vi "Pump Close Selection.vi"(8 "error in (no error)":errorcluster, 11 "Pump Settings In":T1={"Output Device"=enum."Default", "Masterflex"={"VISA resource name"="", "Simulated?"=FALSE, "Pump Number"=0.0, "Reverse?"=FALSE}, "Ismatech"={"VISA resource name"="", "Simulated?"=FALSE, "Pump Number"=0.0, "Reverse?"=FALSE}, "Ismatech 3 Channel Settings"={"VISA resource name"="", "Pump Number"=1, "Channel Number"=0, "Simulated?"=TRUE, "Reverse?"=FALSE}, "VICI Settings"={"VISA resource name"="", "Pump ID"="", "Pump Head Vol"=0.0, "Reverse?"=FALSE, "Simulated?"=FALSE}, "Tacmina Settings"={"Analog DAQ Task"="", "Digital DAQ Task"=""}, "KNF SIMDOS Settings"={"VISA resource name"="", "Simulated?"=FALSE}, "ASIA Pump C"={"ASIA Pump #"=0, "channel"=0, "Simulated"=FALSE}, "FLOM Settings"={"VISA resource name"="", "Simulated?"=FALSE, "Pump Number"=0.0}, "SSI PR/LD Settings"={"VISA resource name"="", "Simulated?"=FALSE}, "SSI P40 Settings"={"VISA resource name"="", "Simulated?"=FALSE}, "Masterflex 75211 Settings"={"Analog DAQ Task"="", "Digital DAQ Task"=""}} {"Ismatech 3 Channel Settings"."Channel Number" min=0 max=3; "Ismatech 3 Channel Settings"."Pump Number" min=1; "Masterflex"."Pump Number" min=1.0 max=20.0 step=1.0; "Ismatech"."Pump Number" min=1.0 max=20.0 step=1.0; "ASIA Pump C"."channel" min=-1 max=1 step=1}) -> (0 "error out":errorcluster, 1 "Connection Error":bool, 3 "Pump Settings Out":T1={"Output Device"=enum."Default", "Masterflex"={"VISA resource name"="", "Simulated?"=FALSE, "Pump Number"=0.0, "Reverse?"=FALSE}, "Ismatech"={"VISA resource name"="", "Simulated?"=FALSE, "Pump Number"=0.0, "Reverse?"=FALSE}, "Ismatech 3 Channel Settings"={"VISA resource name"="", "Pump Number"=1, "Channel Number"=0, "Simulated?"=TRUE, "Reverse?"=FALSE}, "VICI Settings"={"VISA resource name"="", "Pump ID"="", "Pump Head Vol"=0.0, "Reverse?"=FALSE, "Simulated?"=FALSE}, "Tacmina Settings"={"Analog DAQ Task"="", "Digital DAQ Task"=""}, "KNF SIMDOS Settings"={"VISA resource name"="", "Simulated?"=FALSE}, "ASIA Pump C"={"ASIA Pump #"=0, "channel"=0, "Simulated"=FALSE}, "FLOM Settings"={"VISA resource name"="", "Simulated?"=FALSE, "Pump Number"=0.0}, "SSI PR/LD Settings"={"VISA resource name"="", "Simulated?"=FALSE}, "SSI P40 Settings"={"VISA resource name"="", "Simulated?"=FALSE}, "Masterflex 75211 Settings"={"Analog DAQ Task"="", "Digital DAQ Task"=""}} {"Ismatech 3 Channel Settings"."Channel Number" min=0 max=3; "Ismatech 3 Channel Settings"."Pump Number" min=1; "Masterflex"."Pump Number" min=1.0 max=20.0 step=1.0; "Ismatech"."Pump Number" min=1.0 max=20.0 step=1.0; "ASIA Pump C"."channel" min=-1 max=1 step=1})   [LabVIEW 2018, in "Pump Module.lvlib" / "Pump Module Engine.lvlib"]
uses:
  Measure Instrument/Pump Module Engine.lvlib
  Measure Instrument/Pump Settings Cluster.ctl
  Measure Instrument/PID 2 Output Enum.ctl
  Masterflex 7550-30/Controls/Settings Cluster.ctl
  Ismatec ISM 831C/Controls/Ismatech ISM831C Settings Cluster.ctl
  Ismatec 78001/Ismatec 4083.ctl
  VICI M50 Party Mode/Settings Cluster.ctl
  Tacmina QI/Tacmina QI DAQ Setting.ctl
  KNF Pump/Settings Cluster plus SIMDOS.ctl
  ASIA Pump/Pump Settings.ctl
  FLOM Pump/Settings Cluster.ctl
  SSI PR Class/SSI PR or LD Settings Cluster.ctl
  Masterflex 75211/Masterflex 75211 DAQ Setting.ctl
  Ismatec ISM 831C/Ismatec ISM 831C.lvlib
  Masterflex 7550-30/Masterflex 7550-30.lvlib
  VICI M50 Party Mode/VICI M6 M50 Party Mode.lvlib
  Tacmina QI/Tacmina QI.lvlib
  KNF Pump/KNF SIMDOS.lvlib
  ASIA Pump.lvlib
  FLOM Pump/FLOM Pump.lvlib
  SSI PR Class/SSI PR or LD Pump.lvlib
  Masterflex 75211/Masterflex 75211.lvlib
  SSI PR Class/SSI P40 Pump.lvlib
  Pump Module.lvlib
  Ismatec 78001/Ismatec 4308.lvlib
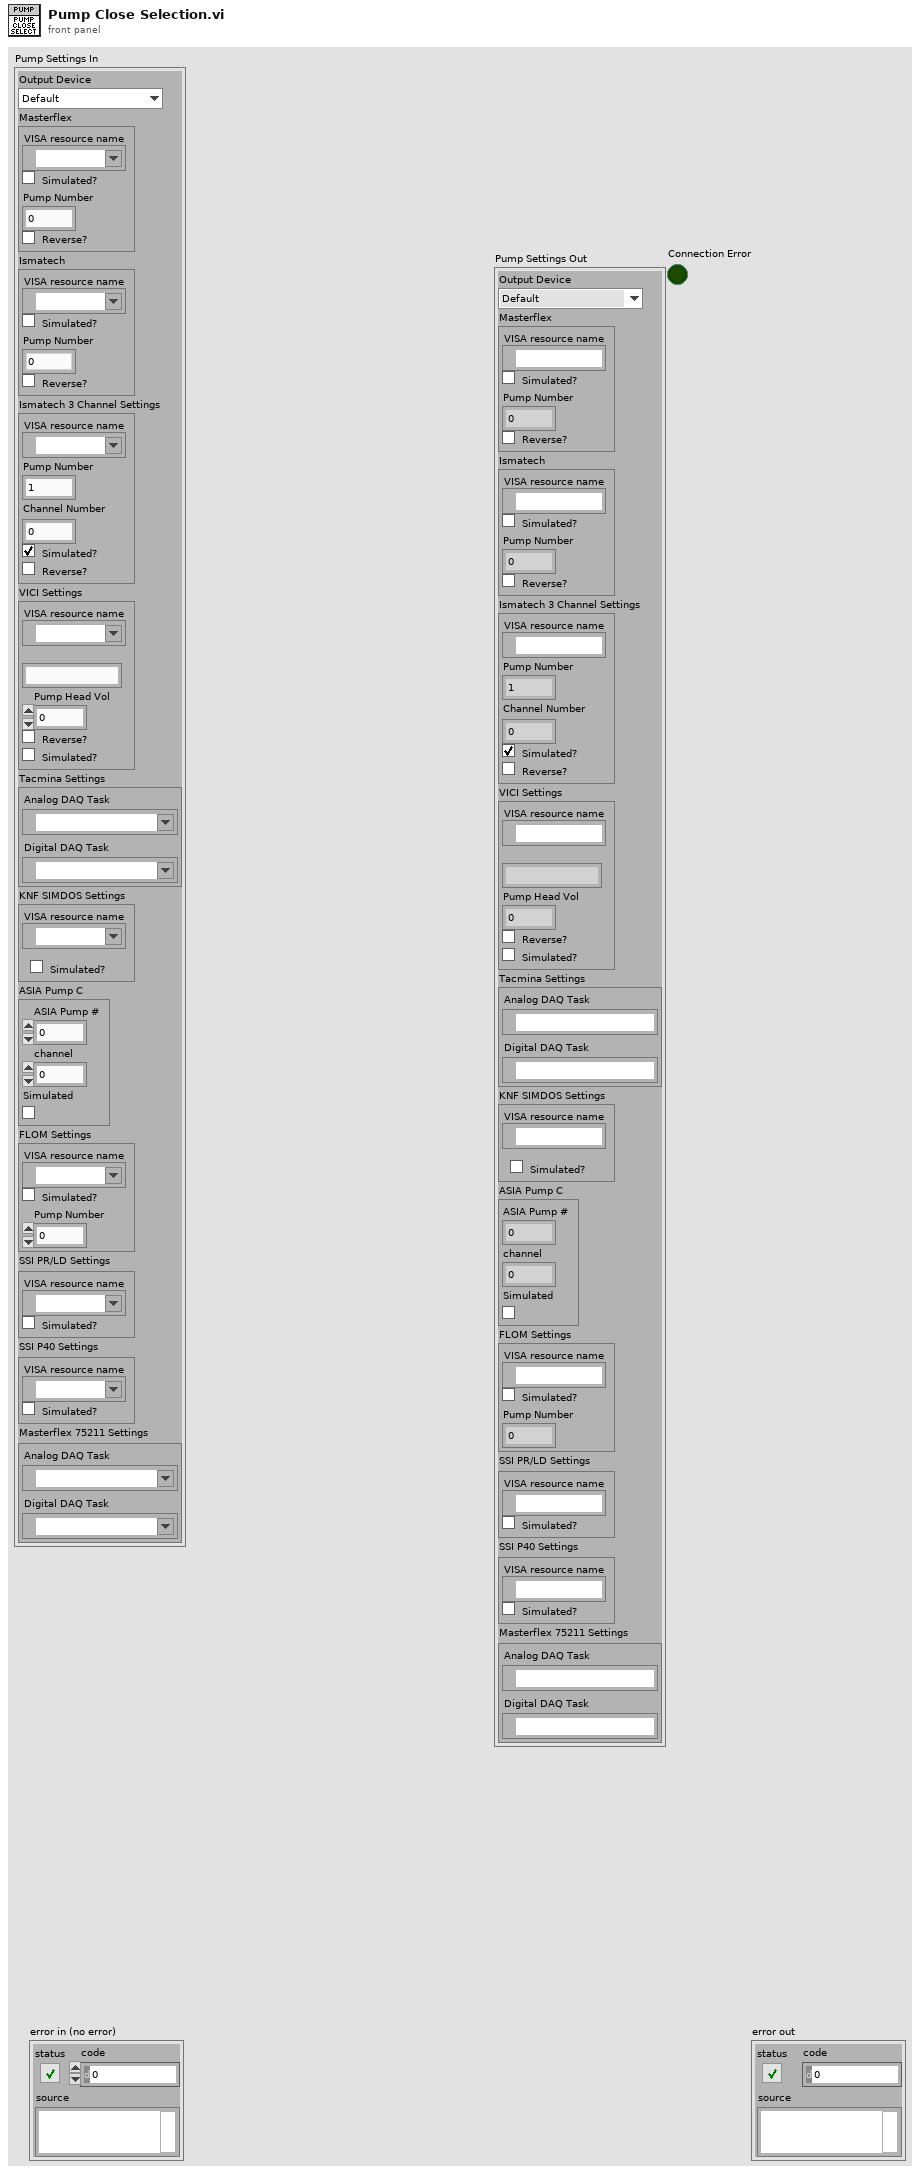
[diagram p1: front panel]
types:
  T1 = typedef "Pump Module.lvlib/Pump Settings Cluster.ctl" = cluster{"Output Device":T2, "Masterflex":T3, "Ismatech":T4, "Ismatech 3 Channel Settings":T5, "VICI Settings":T6, "Tacmina Settings":T7, "KNF SIMDOS Settings":T8, "ASIA Pump C":T9, "FLOM Settings":T10, "SSI PR/LD Settings":T11, "SSI P40 Settings":T11, "Masterflex 75211 Settings":T12}
  T2 = typedef "PID 2 Output Enum.ctl" = enum16{"Default", "Ismatec ISM 4308", "Ismatec ISM 831C", "Masterflex 7550-30", "VICI", "Tacmina QI", "KNF SIMDOS", "ASIA Type C", "FLOM UI-22-11", "SSI PR/LD", "SSI P40", "Masterflex 75211-70"}
  T3 = typedef "Masterflex 7550-30.lvlib/Settings Cluster.ctl" = cluster{"VISA resource name":refnum<visa-resource-name>, "Simulated?":bool, "Pump Number":dbl, "Reverse?":bool}
  T4 = typedef "Ismatec ISM 831C.lvlib/Ismatech ISM831C Settings Cluster.ctl" = cluster{"VISA resource name":refnum<visa-resource-name>, "Simulated?":bool, "Pump Number":dbl, "Reverse?":bool}
  T5 = typedef "Ismatec 4308.lvlib/Ismatec 4083.ctl" = cluster{"VISA resource name":refnum<visa-resource-name>, "Pump Number":i16, "Channel Number":i16, "Simulated?":bool, "Reverse?":bool}
  T6 = typedef "VICI M6 M50 Party Mode.lvlib/Settings Cluster.ctl" = cluster{"VISA resource name":refnum<visa-resource-name>, "Pump ID":string, "Pump Head Vol":dbl, "Reverse?":bool, "Simulated?":bool}
  T7 = typedef "Tacmina QI.lvlib/Tacmina QI DAQ Setting.ctl" = cluster{"Analog DAQ Task":refnum<k21>, "Digital DAQ Task":refnum<k21>}
  T8 = typedef "KNF SIMDOS.lvlib/Settings Cluster plus SIMDOS.ctl" = cluster{"VISA resource name":refnum<visa-resource-name>, "Simulated?":bool}
  T9 = typedef "ASIA Pump.lvlib/Pump Settings.ctl" = cluster{"ASIA Pump #":i32, "channel":i32, "Simulated":bool}
  T10 = typedef "FLOM Pump.lvlib/Settings Cluster.ctl" = cluster{"VISA resource name":refnum<visa-resource-name>, "Simulated?":bool, "Pump Number":dbl}
  T11 = typedef "SSI PR or LD Pump.lvlib/SSI PR or LD Settings Cluster.ctl" = cluster{"VISA resource name":refnum<visa-resource-name>, "Simulated?":bool}
  T12 = typedef "Masterflex 75211.lvlib/Masterflex 75211 DAQ Setting.ctl" = cluster{"Analog DAQ Task":refnum<k21>, "Digital DAQ Task":refnum<k21>}
  T13 = typedef "SSI P40 Pump.lvlib/SSI P40 Settings Cluster.ctl" = cluster{"VISA resource name":refnum<visa-resource-name>, "Simulated?":bool}
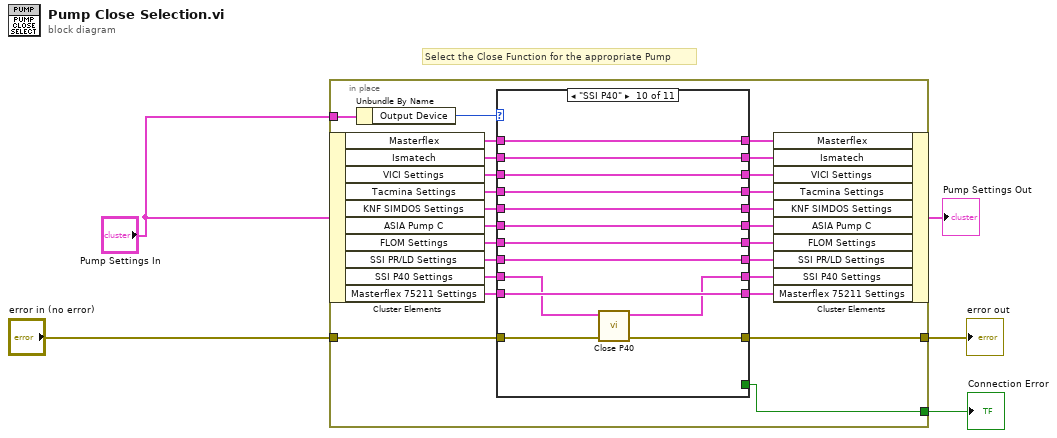
[diagram p0: block diagram]
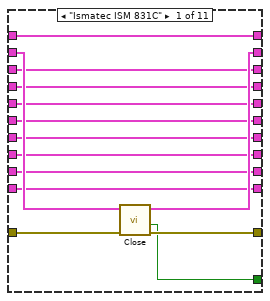
[diagram p2: hidden frame]
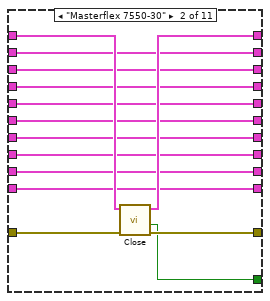
[diagram p3: hidden frame]
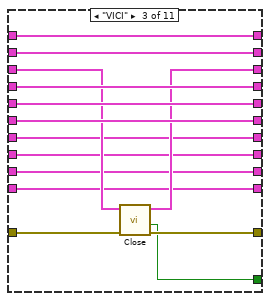
[diagram p4: hidden frame]
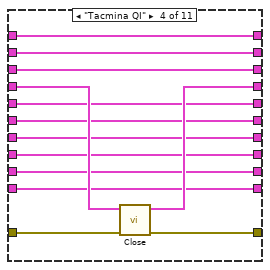
[diagram p5: hidden frame]
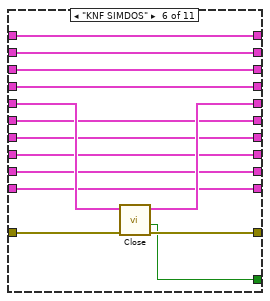
[diagram p7: hidden frame]
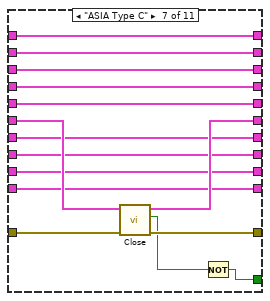
[diagram p8: hidden frame]
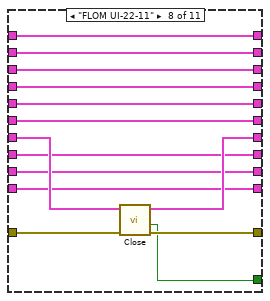
[diagram p9: hidden frame]
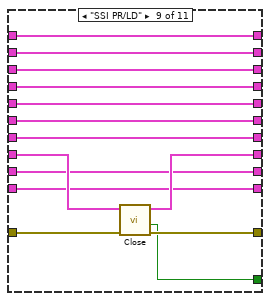
[diagram p10: hidden frame]
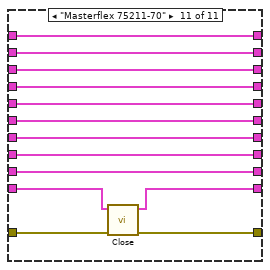
[diagram p11: hidden frame]
diagram:
  # "Select the Close Function for the appropriate Pump"
  n1 = in-place {
    in-place-border: "error in (no error)" -> [w29]
    in-place-border: [w28] -> w4
    in-place-border: "Pump Settings In" -> [w27]
    in-place-border: [w26] -> w3
    n2 = in-place-cluster #1("Pump Settings In") -> ("Masterflex"=w25:T3, "Ismatech"=w24:T4, "VICI Settings"=w23:T6, "Tacmina Settings"=w22:T7, "KNF SIMDOS Settings"=w21:T8, "ASIA Pump C"=w20:T9, "FLOM Settings"=w19:T10, "SSI PR/LD Settings"=w18:T11, "SSI P40 Settings"=w7:T11, "Masterflex 75211 Settings"=w9:T12)
    n3 = Unbundle By Name(w27) -> ("Output Device"=w30:T2)
    n4 = case shown="\"SSI P40\"" w30 {
      tunnel: w25 -> [w40 w58 w69 w82 w96 w110 w123 w139 w153 w165 w178]
      tunnel: [w40 w57 w69 w82 w96 w110 w123 w139 w153 w165 w178] -> w17
      tunnel: w24 -> [w42 w55 w70 w83 w95 w109 w122 w138 w152 w163 w177]
      tunnel: [w44 w56 w71 w84 w94 w106 w124 w132 w145 w164 w169] -> w28
      tunnel: w29 -> [w43 w54 w72 w85 w94 w107 w125 w133 w146 w164 w170]
      tunnel: [w41 w55 w70 w83 w95 w109 w122 w138 w152 w163 w177] -> w16
      tunnel: [w39 w53 w68 w81 w93 w108 w121 w136 w150 w162 w176] -> w14
      tunnel: w22 -> [w39 w53 w68 w80 w93 w108 w121 w136 w150 w162 w176]
      tunnel: [w38 w52 w67 w79 w92 w105 w120 w135 w149 w161 w175] -> w13
      tunnel: w21 -> [w38 w52 w67 w79 w92 w104 w120 w135 w149 w161 w175]
      tunnel: w20 -> [w37 w51 w66 w78 w91 w103 w119 w134 w148 w160 w174]
      tunnel: [w37 w51 w66 w78 w91 w103 w118 w134 w148 w160 w174] -> w12
      tunnel: [w36 w50 w65 w77 w90 w102 w117 w137 w151 w159 w173] -> w15
      tunnel: w23 -> [w36 w50 w64 w77 w90 w102 w117 w137 w151 w159 w173]
      tunnel: [w35 w49 w63 w76 w89 w101 w116 w130 w147 w158 w172] -> w11
      tunnel: w19 -> [w35 w49 w63 w76 w89 w101 w116 w131 w147 w158 w172]
      tunnel: w18 -> [w34 w48 w62 w75 w88 w100 w115 w129 w143 w157 w171]
      tunnel: [w34 w48 w62 w75 w88 w100 w115 w129 w144 w157 w171] -> w10
      tunnel: [w33 w47 w61 _ _ w99 w114 w128 w142 _ _] -> w26
      tunnel: w9 -> [w32 w46 w60 w74 w87 w98 w112 w127 w141 w156 w168]
      tunnel: [w32 w46 w60 w74 w87 w98 w112 w127 w141 w156 w167] -> w8
      tunnel: w7 -> [w31 w45 w59 w73 w86 w97 w111 w126 w140 w155 w166]
      tunnel: [w31 w45 w59 w73 w86 w97 w111 w126 w140 w154 w166] -> w6
      frame "Ismatec ISM 831C" {
        n5 = call "Close.vi"("error in (no error)"=w43, "Ismatech Settings"=w42) -> ("error out"=w44:errorcluster, "Connection Error"=w33:bool, "Ismatech Settings"=w41:T4)  [unwired: 7 in]
      }
      frame "Masterflex 7550-30" {
        n6 = call "Close.vi"("error in (no error)"=w54, "Masterflex Settings in"=w58) -> ("error out"=w56:errorcluster, "Connection Error"=w47:bool, "Masterflex Settings out"=w57:T3)  [unwired: 7 in]
      }
      frame "VICI" {
        n7 = call "Close.vi"("error in (no error)"=w72, "VICI Settings"=w64) -> ("error out"=w71:errorcluster, "Connection Error"=w61:bool, "VICI Settings"=w65:T6)  [unwired: 7 in]
      }
      frame "Tacmina QI" {
        n8 = call "Close.vi"("error in"=w85, "Tacmina Settings in"=w80) -> ("error out"=w84:errorcluster, "Tacmina Settings out"=w81:T7)  [unwired: 8 in]
      }
      frame "Default", Default {
      }
      frame "KNF SIMDOS" {
        n9 = call "Close.vi"("error in (no error)"=w107, "KNF Settings"=w104) -> ("error out"=w106:errorcluster, "Connection Error"=w99:bool, "KNF Settings"=w105:T8)  [unwired: 7 in]
      }
      frame "ASIA Type C" {
        n10 = call "Close.vi"("error in (no error)"=w125, "ASIA Pump C"=w119) -> ("error out"=w124:errorcluster, "Task Completed"=w113:bool, "ASIA Pump C"=w118:T9)  [unwired: 7 in]
        n11 = Not(x=w113) -> (.not. x?=w114:bool)
      }
      frame "FLOM UI-22-11" {
        n12 = call "Close.vi"("error in (no error)"=w133, "FLOM Settings in"=w131) -> ("error out"=w132:errorcluster, "Connection Error"=w128:bool, "FLOM Settings out"=w130:T10)  [unwired: 7 in]
      }
      frame "SSI PR/LD" {
        n13 = call "Close.vi"("error in (no error)"=w146, "SSI PR Settings In"=w143) -> ("error out"=w145:errorcluster, "Connection Error"=w142:bool, "SSI PR Settings Out"=w144:T11)  [unwired: 7 in]
      }
      frame "SSI P40" {
        n14 = call "Close P40.vi"("SSI P40 Settings In"=w155) -> ("SSI P40 Settings Out"=w154:T13)  [unwired: 8 in, 2 out]
      }
      frame "Masterflex 75211-70" {
        n15 = call "Close.vi"("error in"=w170, "Masterflex 75211 Settings"=w168) -> ("error out"=w169:errorcluster, "Masterflex 75211 Settings"=w167:T12)  [unwired: 8 in]
      }
    }
    n16 = in-place-cluster #1("Masterflex"=w17, "Ismatech"=w16, "VICI Settings"=w15, "Tacmina Settings"=w14, "KNF SIMDOS Settings"=w13, "ASIA Pump C"=w12, "FLOM Settings"=w11, "SSI PR/LD Settings"=w10, "SSI P40 Settings"=w6, "Masterflex 75211 Settings"=w8) -> (→"Pump Settings Out":T1)
  }
  "error out" <- w4
  "Connection Error" <- w3
